vi "NotifierGenerate.vi"() -> ()   [LabVIEW 2014]
panel:
  out "GenerateCnt":i32
  in  "stop":bool
  out "32bit integer":i32
  # "Generate"
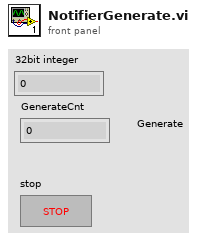
[diagram p1: front panel]
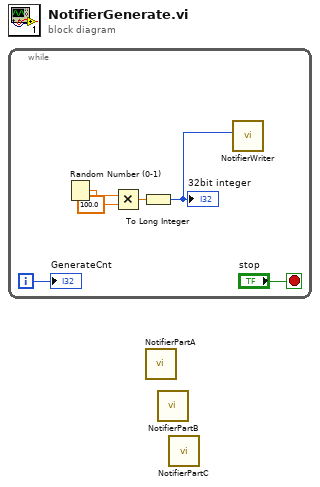
[diagram p0: block diagram]
diagram:
  n1 = while {
    i -> [w1]
    stop <- "stop" stop-if-true
    n2 = Random Number (0-1)() -> (number: 0 to 1=w6:dbl)
    n3 = Multiply(x=w6, y=100.0) -> (x*y=w4:dbl)
    n4 = To Long Integer(number=w4) -> (32bit integer=w3:i32)
    "32bit integer" <- w3
    n5 = call "NotifierWriter.vi"("Numeric"=w3) -> ()  [unwired: 11 in]
    "GenerateCnt" <- w1
  }
  n6 = call "NotifierPartA.vi"() -> ()  [unwired: 12 in]
  n7 = call "NotifierPartB.vi"() -> ()  [unwired: 12 in]
  n8 = call "NotifierPartC.vi"() -> ()  [unwired: 12 in]
